vi "state.vi"() -> ()   [LabVIEW 2020]
panel:
  out "Temp PV":dbl format="%#.1f"
  out "Waveform Chart":dbl(graph)
  out "x-y":dbl
  out "Power LED":bool
  in  "Temp SV":dbl=120.0
  in  "Time":dbl=300.0
  in  "Stop Button":bool
  in  "Play Button":bool
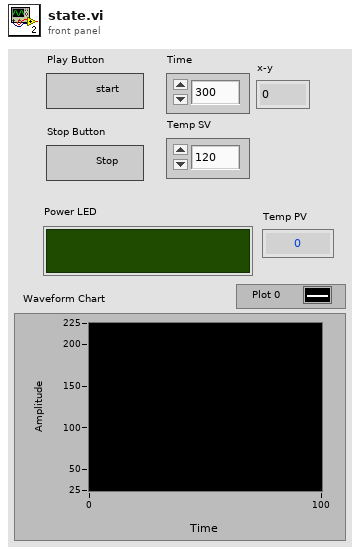
[diagram p1: front panel]
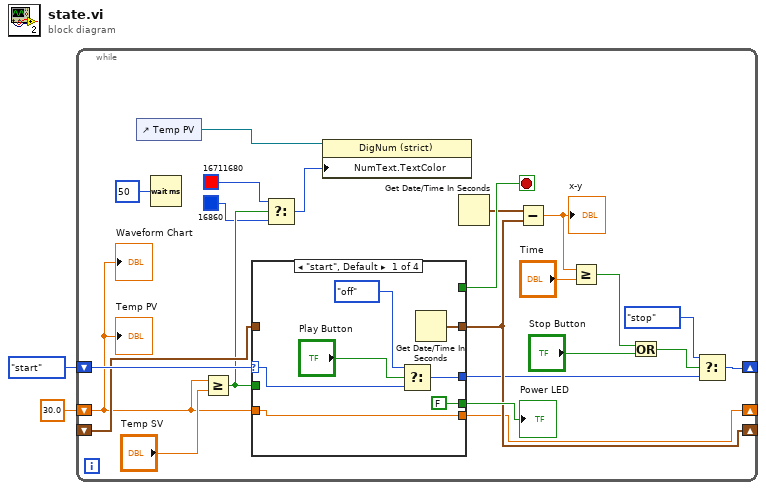
[diagram p0: block diagram]
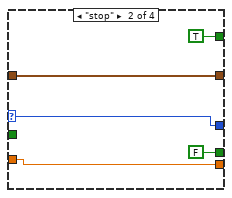
[diagram p2: hidden frame]
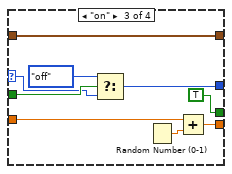
[diagram p3: hidden frame]
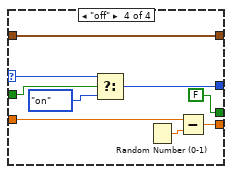
[diagram p4: hidden frame]
diagram:
  n1 = while {
    shift-right: [w13] -> _
    shift-left: enum16{"start", "stop", "on", "off"}."start" -> [w25]
    shift-right: [w19] -> _
    shift-left: _ -> [w21]
    shift-right: [w10] -> _
    shift-left: 30.0 -> [w9]
    stop <- w22 stop-if-true
    n2 = control-ref of="Temp PV"() -> (w4:refnum<vi>)
    n3 = Wait (ms)(milliseconds to wait=u32 50) -> ()  [unwired: 1 out]
    n4 = Greater Or Equal?(x=w9, y="Temp SV") -> (x >= y?=w7:bool)
    n5 = case shown="\"start\", Default" w25 {
      selector: w25 -> [w31 w36 w44 w52]
      tunnel: [w30 w36 w42 w54] -> w15
      tunnel: [FALSE FALSE TRUE FALSE] -> w24
      tunnel: w7 -> [_ _ w45 w53]
      tunnel: [_ TRUE _ _] -> w22
      tunnel: [w27 w34 w41 w50] -> w19
      tunnel: w21 -> [_ w34 w41 w50]
      tunnel: w9 -> [w26 w33 w40 w49]
      tunnel: [w26 w33 w38 w47] -> w10
      frame "start", Default {
        n6 = Select(t=enum16{"start", "stop", "on", "off"}."off", s="Play Button", f=w31) -> (s? t:f=w30:enum16{"start", "stop", "on", "off"})
        n7 = Get Date/Time In Seconds() -> (seconds since 1Jan1904=w27:timestamp)
      }
      frame "stop" {
      }
      frame "on" {
        n8 = Select(t=enum16{"start", "stop", "on", "off"}."off", s=w45, f=w44) -> (s? t:f=w42:enum16{"start", "stop", "on", "off"})
        n9 = Random Number (0-1)() -> (number: 0 to 1=w39:dbl)
        n10 = Add(x=w40, y=w39) -> (x+y=w38:dbl)
      }
      frame "off" {
        n11 = Select(t=w52, s=w53, f=enum16{"start", "stop", "on", "off"}."on" ("t")) -> (s? t:f=w54:enum16{"start", "stop", "on", "off"})
        n12 = Random Number (0-1)() -> (number: 0 to 1=w48:dbl)
        n13 = Subtract(x=w49, y=w48) -> (x-y=w47:dbl)
      }
    }
    "Power LED" <- w24
    n14 = Select(t=u32 16711680 ("Numeric Text.Text Colors:Text Color"), s=w7, f=u32 16860 ("Numeric Text.Text Colors:Text Color")) -> (s? t:f=w3:u32)
    n15 = property class="DigNum (strict)"(reference=w4, "NumText.TextColor"=w3) -> ()  [unwired: 1 in, 2 out]
    n16 = Get Date/Time In Seconds() -> (seconds since 1Jan1904=w20:timestamp)
    n17 = Subtract(x=w20, y=w19) -> (x-y=w18:dbl)
    "x-y" <- w18
    n18 = Greater Or Equal?(x=w18, y="Time") -> (x >= y?=w16:bool)
    n19 = Or(x=w16, y="Stop Button") -> (x .or. y?=w12:bool)
    n20 = Select(t=enum16{"start", "stop", "on", "off"}."stop", s=w12, f=w15) -> (s? t:f=w13:enum16{"start", "stop", "on", "off"})
    "Waveform Chart" <- w9
    "Temp PV" <- w9
  }
